vi "CLD 11 Producer consumer events solution.vi"() -> ()   [LabVIEW 2009]
doc: "CLD-Übung 11\n\nIn diesem VI wird eine Erzeuger/Verbraucher-Architektur mit einer Ereignisstruktur verwendet. Da nur ein Datenwert (Zielzeit) genutzt werden kann, werden Änderungen für das Element \"Zielzeit\" mit Hilfe von Polling und nicht mit einer Ereignisstruktur überwacht."
uses:
  CLD 11 producer consumer enum.ctl
  CLD 11 CSV file enum.ctl
  CLD 11 CSV file data structure.ctl
  CLD 11 Producer Consumer Data Structure.ctl
panel:
  out "Aktuelle Zielzeit":dbl
  out "Verstrichene Zeit (s)":dbl
  out "Schritt 3":bool
  out "Schritt 2":bool
  out "Schritt 1":bool
  out "Zeit ist verstrichen":bool
  in  "Autom. zurücksetzen":bool
  in  "Zurücksetzen-Schaltfläche":bool
  in  "VI anhalten":bool
  in  "Zielzeit (s)":dbl
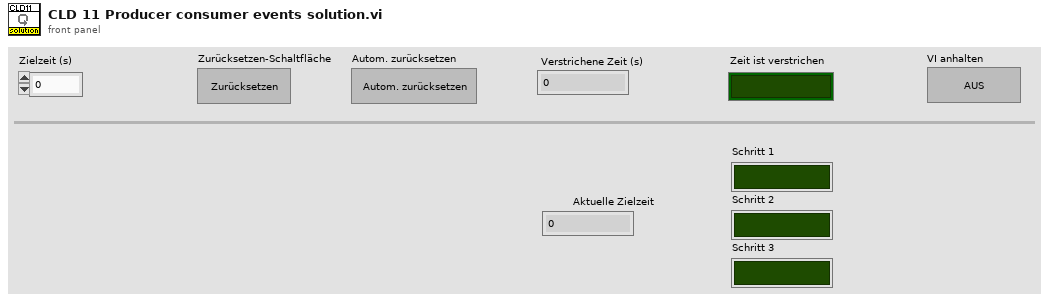
[diagram p1: front panel]
types:
  T1 = typedef "CLD 11 Producer Consumer Data Structure.ctl" = cluster{"Datenstruktur der CSV-Datei":T2, "Zeit ist verstrichen":bool, "Zurücksetzen":bool, "Autom. zurücksetzten":bool, "Zielzeit (s)":dbl, "Nr. des aktuellen Zustands":i32}
  T2 = typedef "CLD 11 CSV file data structure.ctl" = cluster{"Verweildauer":i32, "Zustand 1":bool, "Zustand 2":bool, "Zustand 3":bool}
  T3 = typedef "CLD 11 producer consumer enum.ctl" = enum16{"App initialisieren", "CSV-Datei lesen", "Timer prüfen", "Zustand 1 ausführen", "Zustand 2 ausführen", "Zustand 3 ausführen", "App anhalten", "Zurücksetzen", "Autom. zurücksetzten"}
  T4 = typedef "CLD 11 CSV file enum.ctl" = enum16{"CSV lesen", "CSV schreiben"}
  T5 = cluster{"Status":bool, "Code":i32, "Quelle":string}
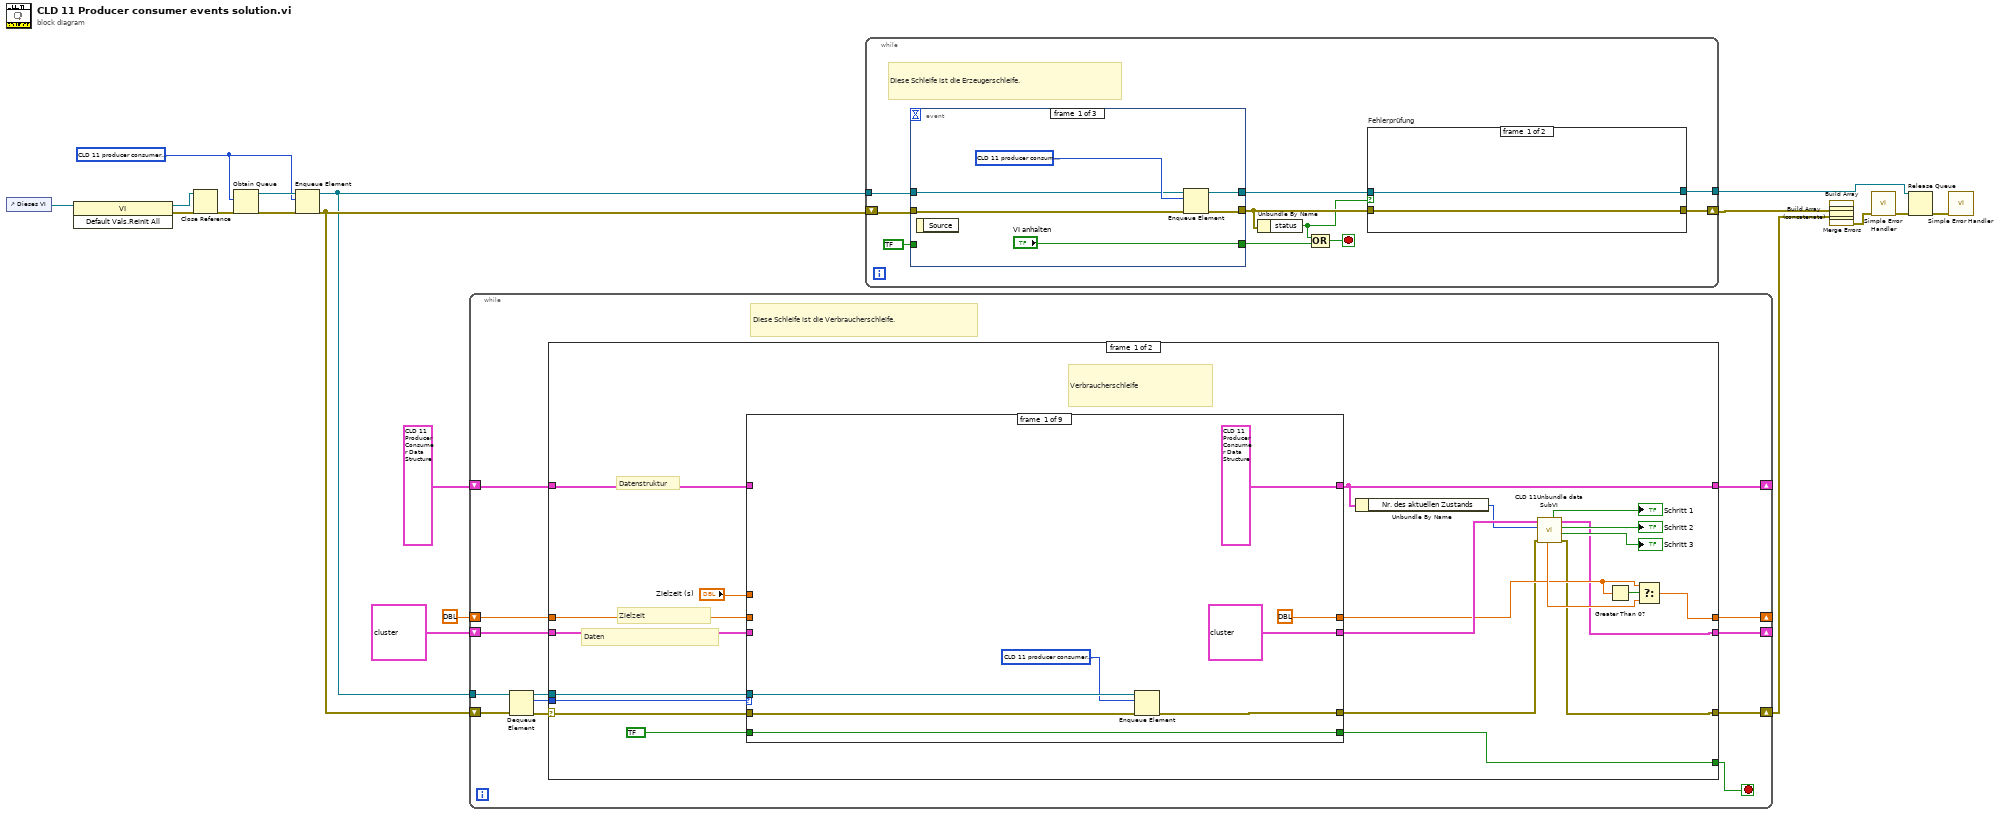
[diagram p0: block diagram]
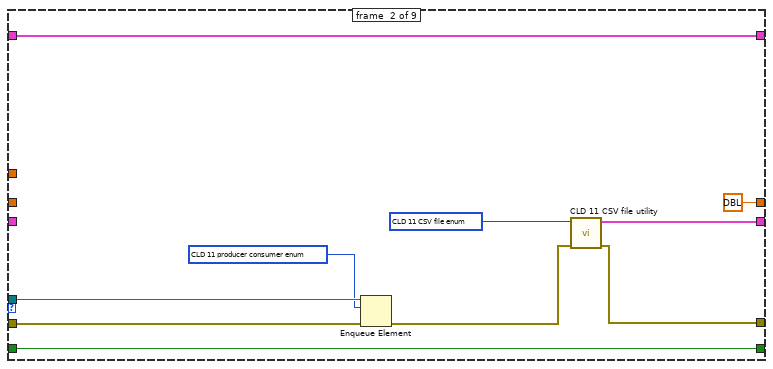
[diagram p2: hidden frame]
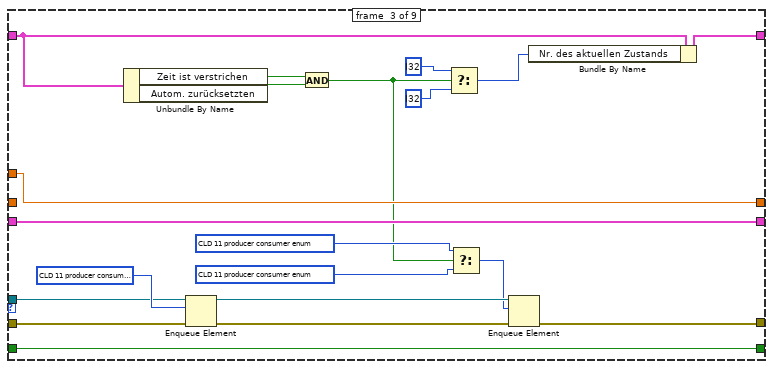
[diagram p3: hidden frame]
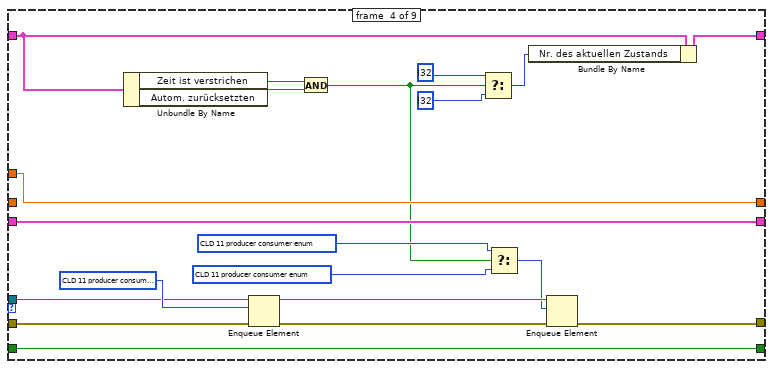
[diagram p4: hidden frame]
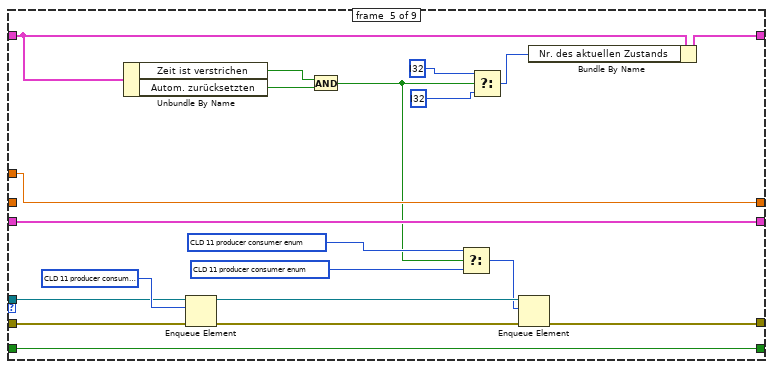
[diagram p5: hidden frame]
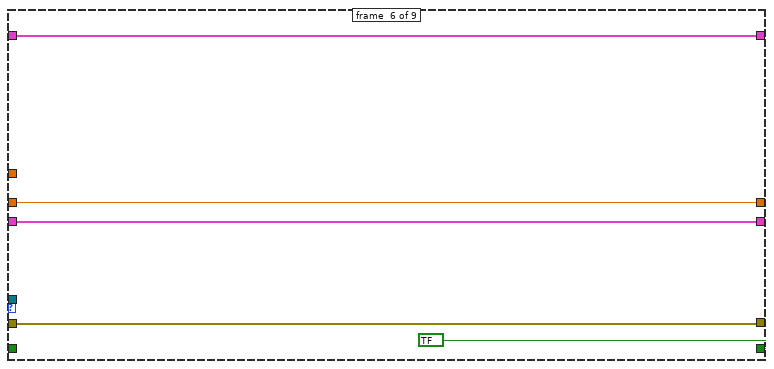
[diagram p6: hidden frame]
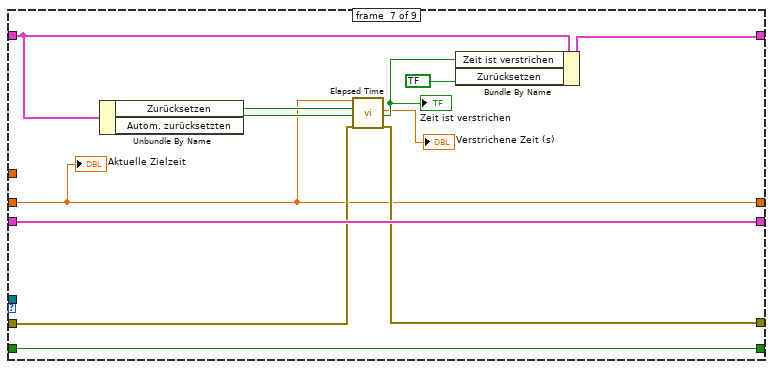
[diagram p7: hidden frame]
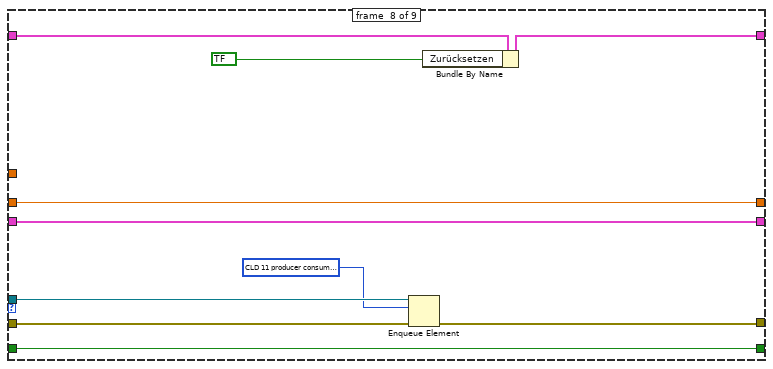
[diagram p8: hidden frame]
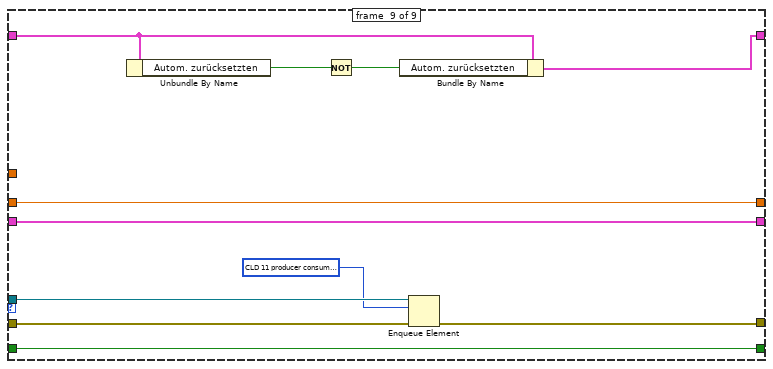
[diagram p9: hidden frame]
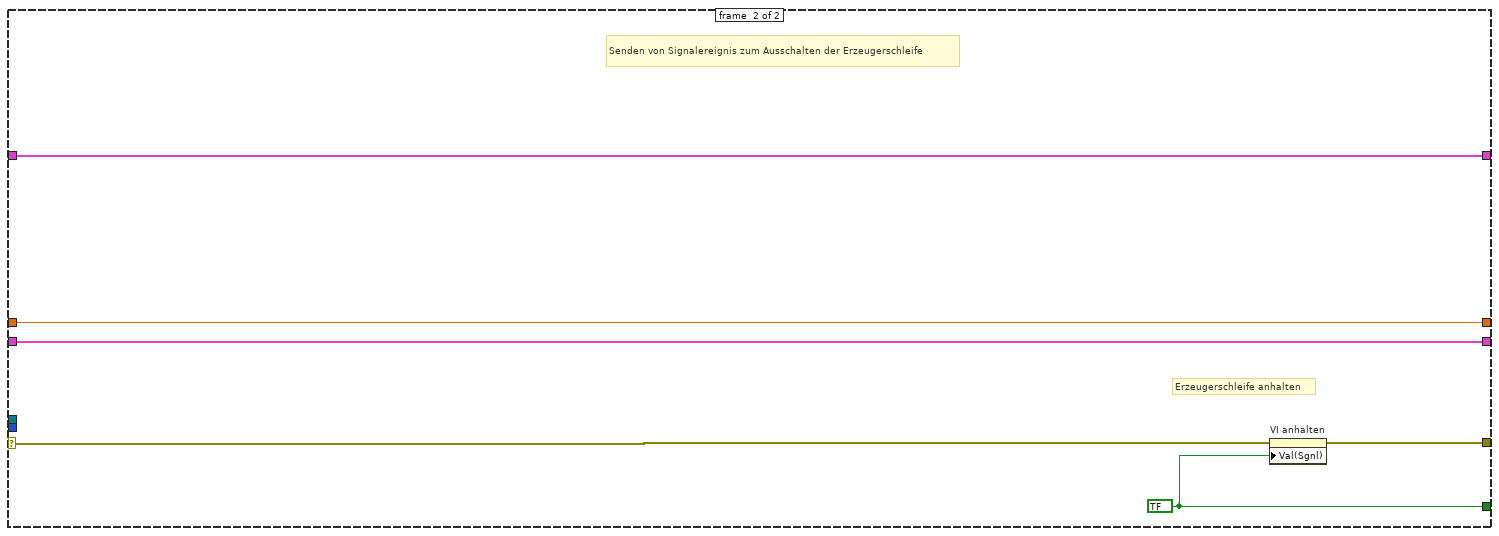
[diagram p10: hidden frame]
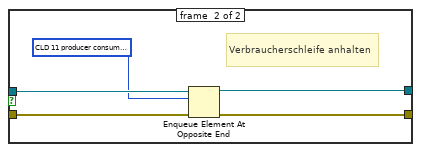
[diagram p11: hidden frame]
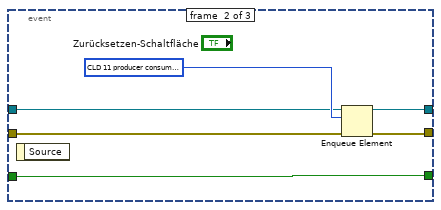
[diagram p12: hidden frame]
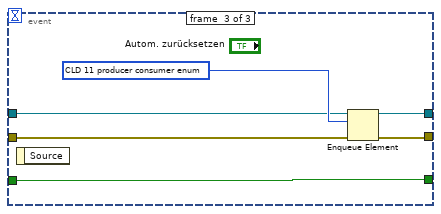
[diagram p13: hidden frame]
diagram:
  w13 = T3 ? ("Enum für Timer 1 in CLD 8")
  n1 = control-ref of="Dieses VI"() -> (w19:refnum<vi>)
  n2 = invoke on="Invoke Node" class="VI" method="Default Vals.Reinit All"(reference=w19) -> (reference out=w17:refnum<vi>, error out=w18:errorcluster)  [unwired: 2 in, 1 out]
  n3 = Close Reference(reference=w17, error in (no error)=w18) -> (error out=w16:errorcluster)
  n4 = Obtain Queue(element data type=w13, error in (no error)=w16) -> (queue out=w20:refnum<queue>, error out=w15:errorcluster)  [unwired: 3 in, 1 out]
  n5 = Enqueue Element(queue=w20, element=w13, error in (no error)=w15) -> (queue out=w7:refnum<queue>, error out=w14:errorcluster)  [unwired: 1 in, 1 out]
  n6 = while {
    tunnel: w7 -> [w33]
    shift-right: [w28] -> w3
    shift-left: w14 -> [w27]
    shift-right: [w26] -> _
    shift-left: T2[] ? ("[Daten, Ausgang]") -> [w25]
    shift-right: [w24] -> _
    shift-left: dbl ? -> [w23]
    shift-right: [w22] -> _
    shift-left: T1 ? ("Erzeuger/Verbraucher-Datenstruktur") -> [w21]
    stop <- w30 stop-if-true
    # "Diese Schleife ist die Verbraucherschleife."
    n7 = Dequeue Element(queue=w33, error in (no error)=w27) -> (queue out=w29:refnum<queue>, element=w31:T3, error out=w32:errorcluster)  [unwired: 1 in, 1 out]
    n8 = case shown="Error" w32 {
      selector: w32 -> [w51 w172]
      tunnel: w31 -> [w53 _]
      tunnel: [w55 w174] -> w30
      tunnel: w29 -> [w52 _]
      tunnel: [w36 w173] -> w28
      tunnel: [w34 w176] -> w26
      tunnel: w25 -> [w50 w176]
      tunnel: [w42 w177] -> w24
      tunnel: w23 -> [w49 w177]
      tunnel: [w41 w175] -> w22
      tunnel: w21 -> [w48 w175]
      frame #0 {
        # "Daten"
        # "Zielzeit"
        # "Datenstruktur"
        # "Verbraucherschleife"
        n9 = case shown="\"Autom. zurücksetzten\"" w53 {
          tunnel: [w63 w73 w93 w113 w133 bool ? w150 w160 w171] -> w55
          tunnel: bool ? -> [w63 w73 w93 w113 w133 _ w150 w160 w171]
          tunnel: w52 -> [w60 w71 w90 w110 w130 _ _ w155 w168]
          tunnel: w51 -> [w62 w72 w88 w108 w128 w135 w148 w154 w167]
          tunnel: [w61 w66 w86 w106 w126 w135 w147 w153 w166] -> w37
          tunnel: [T2[] ? ("[Daten, Ausgang]") w69 w92 w112 w132 w138 w149 w159 w170] -> w44
          tunnel: w50 -> [_ _ w92 w112 w132 w138 w149 w159 w170]
          tunnel: [dbl ? dbl ? ("Verweildauer") w81 w101 w122 w137 w140 w151 w164] -> w43
          tunnel: w49 -> [_ _ _ _ _ w137 w140 w151 w164]
          tunnel: [T1 ? ("Erzeuger/Verbraucher-Datenstruktur") w64 w80 w100 w121 w136 w145 w158 w169] -> w41
          tunnel: w48 -> [_ w64 w85 w105 w125 w136 w144 w157 w163]
          tunnel: "Zielzeit (s)" -> [_ _ w81 w101 w122 _ _ _ _]
          frame #0 {
            n10 = Enqueue Element(queue=w60, element=T3 ? ("Enum für Timer 1 in CLD 8"), error in (no error)=w62) -> (error out=w61:errorcluster)  [unwired: 1 in, 2 out]
          }
          frame #1 {
            n11 = Enqueue Element(queue=w71, element=T3 ? ("Enum für Timer 1 in CLD 8"), error in (no error)=w72) -> (error out=w67:errorcluster)  [unwired: 1 in, 2 out]
            n12 = call "CLD 11 CSV file utility.vi"("Fehler (Eingang)"=w67, "CSV-Datei-Enum"=T4 ?) -> ("Fehler (Ausgang)"=w66:T5, "[Daten, Ausgang]"=w69:T2[])  [unwired: 8 in]
          }
          frame #2 {
            n13 = Unbundle By Name(w85) -> ("Zeit ist verstrichen"=w75:bool, "Autom. zurücksetzten"=w76:bool)
            n14 = Enqueue Element(queue=w90, element=T3 ? ("Enum für Timer 1 in CLD 8"), error in (no error)=w88) -> (queue out=w89:refnum<queue>, error out=w87:errorcluster)  [unwired: 1 in, 1 out]
            n15 = And(x=w75, y=w76) -> (x .and. y?=w74:bool)
            n16 = Select(t=i32 ? ("Nr. des aktuellen Zustands"), s=w74, f=i32 ? ("Nr. des aktuellen Zustands")) -> (s? t:f=w77:i32)
            n17 = Select(t=T3 ? ("Enum für Timer 1 in CLD 8"), s=w74, f=T3 ? ("Enum für Timer 1 in CLD 8")) -> (s? t:f=w82:T3)
            n18 = Enqueue Element(queue=w89, element=w82, error in (no error)=w87) -> (error out=w86:errorcluster)  [unwired: 1 in, 2 out]
            n19 = Bundle By Name(cluster=w85, "Nr. des aktuellen Zustands"=w77) -> (w80:T1)
          }
          frame #3 {
            n20 = Unbundle By Name(w105) -> ("Zeit ist verstrichen"=w95:bool, "Autom. zurücksetzten"=w96:bool)
            n21 = Enqueue Element(queue=w110, element=T3 ? ("Enum für Timer 1 in CLD 8"), error in (no error)=w108) -> (queue out=w109:refnum<queue>, error out=w107:errorcluster)  [unwired: 1 in, 1 out]
            n22 = And(x=w95, y=w96) -> (x .and. y?=w94:bool)
            n23 = Select(t=i32 ? ("Nr. des aktuellen Zustands"), s=w94, f=i32 ? ("Nr. des aktuellen Zustands")) -> (s? t:f=w97:i32)
            n24 = Select(t=T3 ? ("Enum für Timer 1 in CLD 8"), s=w94, f=T3 ? ("Enum für Timer 1 in CLD 8")) -> (s? t:f=w102:T3)
            n25 = Bundle By Name(cluster=w105, "Nr. des aktuellen Zustands"=w97) -> (w100:T1)
            n26 = Enqueue Element(queue=w109, element=w102, error in (no error)=w107) -> (error out=w106:errorcluster)  [unwired: 1 in, 2 out]
          }
          frame #4 {
            n27 = Unbundle By Name(w125) -> ("Zeit ist verstrichen"=w115:bool, "Autom. zurücksetzten"=w116:bool)
            n28 = Enqueue Element(queue=w130, element=T3 ? ("Enum für Timer 1 in CLD 8"), error in (no error)=w128) -> (queue out=w129:refnum<queue>, error out=w127:errorcluster)  [unwired: 1 in, 1 out]
            n29 = And(x=w115, y=w116) -> (x .and. y?=w114:bool)
            n30 = Select(t=T3 ? ("Enum für Timer 1 in CLD 8"), s=w114, f=T3 ? ("Enum für Timer 1 in CLD 8")) -> (s? t:f=w123:T3)
            n31 = Select(t=i32 ? ("Nr. des aktuellen Zustands"), s=w114, f=i32 ? ("Nr. des aktuellen Zustands")) -> (s? t:f=w118:i32)
            n32 = Enqueue Element(queue=w129, element=w123, error in (no error)=w127) -> (error out=w126:errorcluster)  [unwired: 1 in, 2 out]
            n33 = Bundle By Name(cluster=w125, "Nr. des aktuellen Zustands"=w118) -> (w121:T1)
          }
          frame #5 {
          }
          frame #6 {
            n34 = Unbundle By Name(w144) -> ("Zurücksetzen"=w143:bool, "Autom. zurücksetzten"=w142:bool)
            n35 = call "Elapsed Time"("Time Target (s)"=w140, "Reset"=w143, "Auto Reset"=w142, "error in (no error)"=w148) -> ("Elapsed Time (s)"=→"Verstrichene Zeit (s)":dbl, "Time has Elapsed"=w146:bool, "error out"=w147:errorcluster)  [unwired: 8 in, 5 out]
            "Zeit ist verstrichen" <- w146
            n36 = Bundle By Name(cluster=w144, "Zeit ist verstrichen"=w146, "Zurücksetzen"=bool ?) -> (w145:T1)
            "Aktuelle Zielzeit" <- w140
          }
          frame #7 {
            n37 = Enqueue Element(queue=w155, element=T3 ? ("Element"), error in (no error)=w154) -> (error out=w153:errorcluster)  [unwired: 1 in, 2 out]
            n38 = Bundle By Name(cluster=w157, "Zurücksetzen"=bool ?) -> (w158:T1)
          }
          frame #8 {
            n39 = Unbundle By Name(w163) -> ("Autom. zurücksetzten"=w162:bool)
            n40 = Not(x=w162) -> (.not. x?=w161:bool)
            n41 = Bundle By Name(cluster=w163, "Autom. zurücksetzten"=w161) -> (w169:T1)
            n42 = Enqueue Element(queue=w168, element=T3 ? ("Element"), error in (no error)=w167) -> (error out=w166:errorcluster)  [unwired: 1 in, 2 out]
          }
        }
        n43 = Unbundle By Name(w41) -> ("Nr. des aktuellen Zustands"=w40:i32)
        n44 = call "CLD 11Unbundle data SubVI.vi"("Fehler (Eingang, kein Fehler)"=w37, "Nr. des aktuellen Zustands"=w40, "[Daten, Eingang]"=w44) -> ("Fehler (Ausgang)"=w36:errorcluster, "Zustand 3"=→"Schritt 3":bool, "Zustand 2"=→"Schritt 2":bool, "[Daten, Ausgang]"=w34:T2[], "Zustand 1"=→"Schritt 1":bool, "Verweildauer"=w46:dbl)  [unwired: 2 in, 1 out]
        n45 = Greater Than 0?(x=w43) -> (x > 0?=w45:bool)
        n46 = Select(t=w43, s=w45, f=w46) -> (s? t:f=w42:dbl)
      }
      frame #1 {
        w174 = bool ?
        # "Erzeugerschleife anhalten"
        # "Senden von Signalereignis zum Ausschalten der Erzeugerschleife"
        n47 = property on="VI anhalten" class="Bool (strict)"(error in=w172, "Val(Sgnl)"=w174) -> (error out=w173:errorcluster)  [unwired: 1 in, 1 out]
      }
    }
  }
  n48 = while {
    tunnel: w7 -> [w187]
    tunnel: [w178] -> w6
    shift-right: [w183] -> w4
    shift-left: w14 -> [w186]
    stop <- w179 stop-if-true
    # "Diese Schleife ist die Erzeugerschleife."
    n49 = event shown="[1] \"Zurücksetzen-Schaltfläche\": Value Change" {
      selector: _ -> [_ _ _]
      dyn-events: _ -> [_ _ _]
      timeout: _ -> [_ _ _]
      tunnel: w187 -> [w196 w203 w209]
      tunnel: w186 -> [w199 w206 w212]
      tunnel: [w198 w205 w211] -> w181
      tunnel: ["VI anhalten" w202 w208] -> w185
      tunnel: bool ? ("VI anhalten") -> [_ w202 w208]
      tunnel: [w195 w201 w207] -> w182
      event #0 {
        n50 = event-data() -> ()  [unwired: 1 in, 1 out]
        n51 = Enqueue Element(queue=w196, element=T3 ? ("Enum für Timer 1 in CLD 8"), error in (no error)=w199) -> (queue out=w195:refnum<queue>, error out=w198:errorcluster)  [unwired: 1 in, 1 out]
      }
      event #1 {
        n52 = event-data() -> ()  [unwired: 1 in, 1 out]
        n53 = Enqueue Element(queue=w203, element=T3 ? ("Enum für Timer 1 in CLD 8"), error in (no error)=w206) -> (queue out=w201:refnum<queue>, error out=w205:errorcluster)  [unwired: 1 in, 1 out]
      }
      event #2 {
        n54 = event-data() -> ()  [unwired: 1 in, 1 out]
        n55 = Enqueue Element(queue=w209, element=T3 ? ("Enum für Timer 1 in CLD 8"), error in (no error)=w212) -> (queue out=w207:refnum<queue>, error out=w211:errorcluster)  [unwired: 1 in, 1 out]
      }
    }
    n56 = Unbundle By Name(w181) -> ("status"=w180:bool)
    n57 = Compound Arithmetic op=OR(w180, w185) -> (w179:bool)
    n58 = case "Fehlerprüfung" shown="True" w180 {
      tunnel: w181 -> [w189 w191]
      tunnel: [w189 w190] -> w183
      tunnel: w182 -> [w188 w194]
      tunnel: [w188 w192] -> w178
      frame #0 {
      }
      frame #1 {
        # "Verbraucherschleife anhalten"
        n59 = Enqueue Element At Opposite End(queue=w194, element=T3 ? ("Enum für Timer 1 in CLD 8"), error in (no error)=w191) -> (queue out=w192:refnum<queue>, error out=w190:errorcluster)  [unwired: 1 in, 1 out]
      }
    }
  }
  n60 = Build Array(w4, w3) -> (w2:errorcluster[])
  n61 = Build Array (concatenate)(w2) -> (w1:errorcluster[])
  n62 = call <vilib>:"Merge Errors.vi"("error array in"=w1) -> ("error out"=w5:errorcluster)  [unwired: 6 in]
  n63 = call <vilib>:"Simple Error Handler.vi"("error in (no error)"=w5) -> ("error out"=w12:errorcluster)  [unwired: 4 in, 4 out]
  n64 = Release Queue(queue=w6, error in (no error)=w12) -> (error out=w8:errorcluster)  [unwired: 1 in, 2 out]
  n65 = call <vilib>:"Simple Error Handler.vi"("error in (no error)"=w8) -> ()  [unwired: 4 in, 5 out]
